vi "系统设置.vi"() -> ()   [LabVIEW 2016]
uses:
  <vilib>/Utility/miscctls.llb/LVPointTypeDef.ctl
  <vilib>/ptbypt/NI_PtbyPt.lvlib
  <vilib>/Utility/config.llb/NI_LVConfig.lvlib
panel:
  in  "多参数运行间隔":i16=4 min=0 max=24
  out "最近一次启动时间":string
  in  "站点信息设置":bool
  in  "定时重启配置":bool
  in  "模块启用配置":bool
  in  "首页显示设置":bool
  in  "开机启动":bool caption="氨氮禁用"
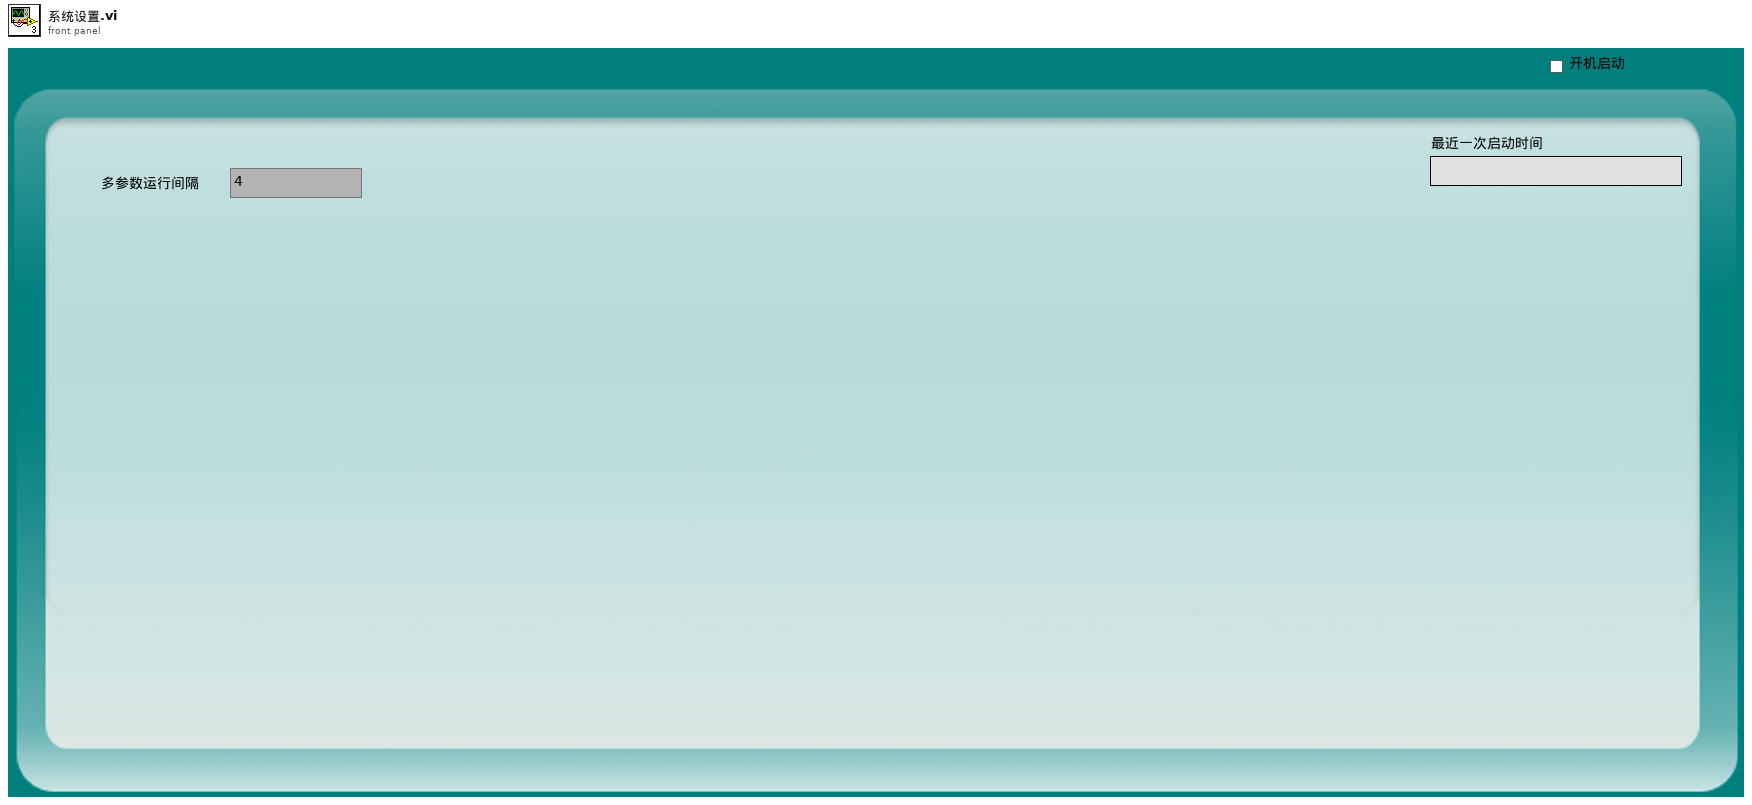
[diagram p1: front panel]
types:
  T1 = typedef "参数.ctl" = cluster{"测试模式":enum16{"水样测试", "平行样测试", "集成干预测试", "加标回收"}, "参数启用":T2}
  T2 = typedef "启动参数.ctl" = cluster{"氨氮":bool, "总磷":bool, "总氮":bool, "多参数":bool, "CODmn":bool, "CODCr":bool, "氟化物":bool, "超标留样":bool, "重金属":bool, "挥发酚":bool}
  T3 = typedef "LVPointTypeDef.ctl" = cluster{"Horizontal":i16, "Vertical":i16}
  T4 = enum8{"Enabled", "Disabled", "Disabled and Grayed Out"}
  T5 = cluster{"频次":enum16{"关闭", "每天", "星期一", "星期二", "星期三", "星期四", "星期五", "星期六", "星期日"}, "时":u16, "分":u16}
  T6 = typedef "LVDateTimeRec.ctl" = cluster{"秒数的小数部分":dbl, "秒":i32, "分":i32, "时":i32, "日":i32, "月":i32, "年":i32, "天数（周）":i32, "天数（年）":i32, "DST":i32}
  T7 = enum16{"关闭", "每天", "星期一", "星期二", "星期三", "星期四", "星期五", "星期六", "星期日"}
  T8 = typedef "NI_LVConfig.lvlib/Config Data RefNum.ctl" = refnum<k1>
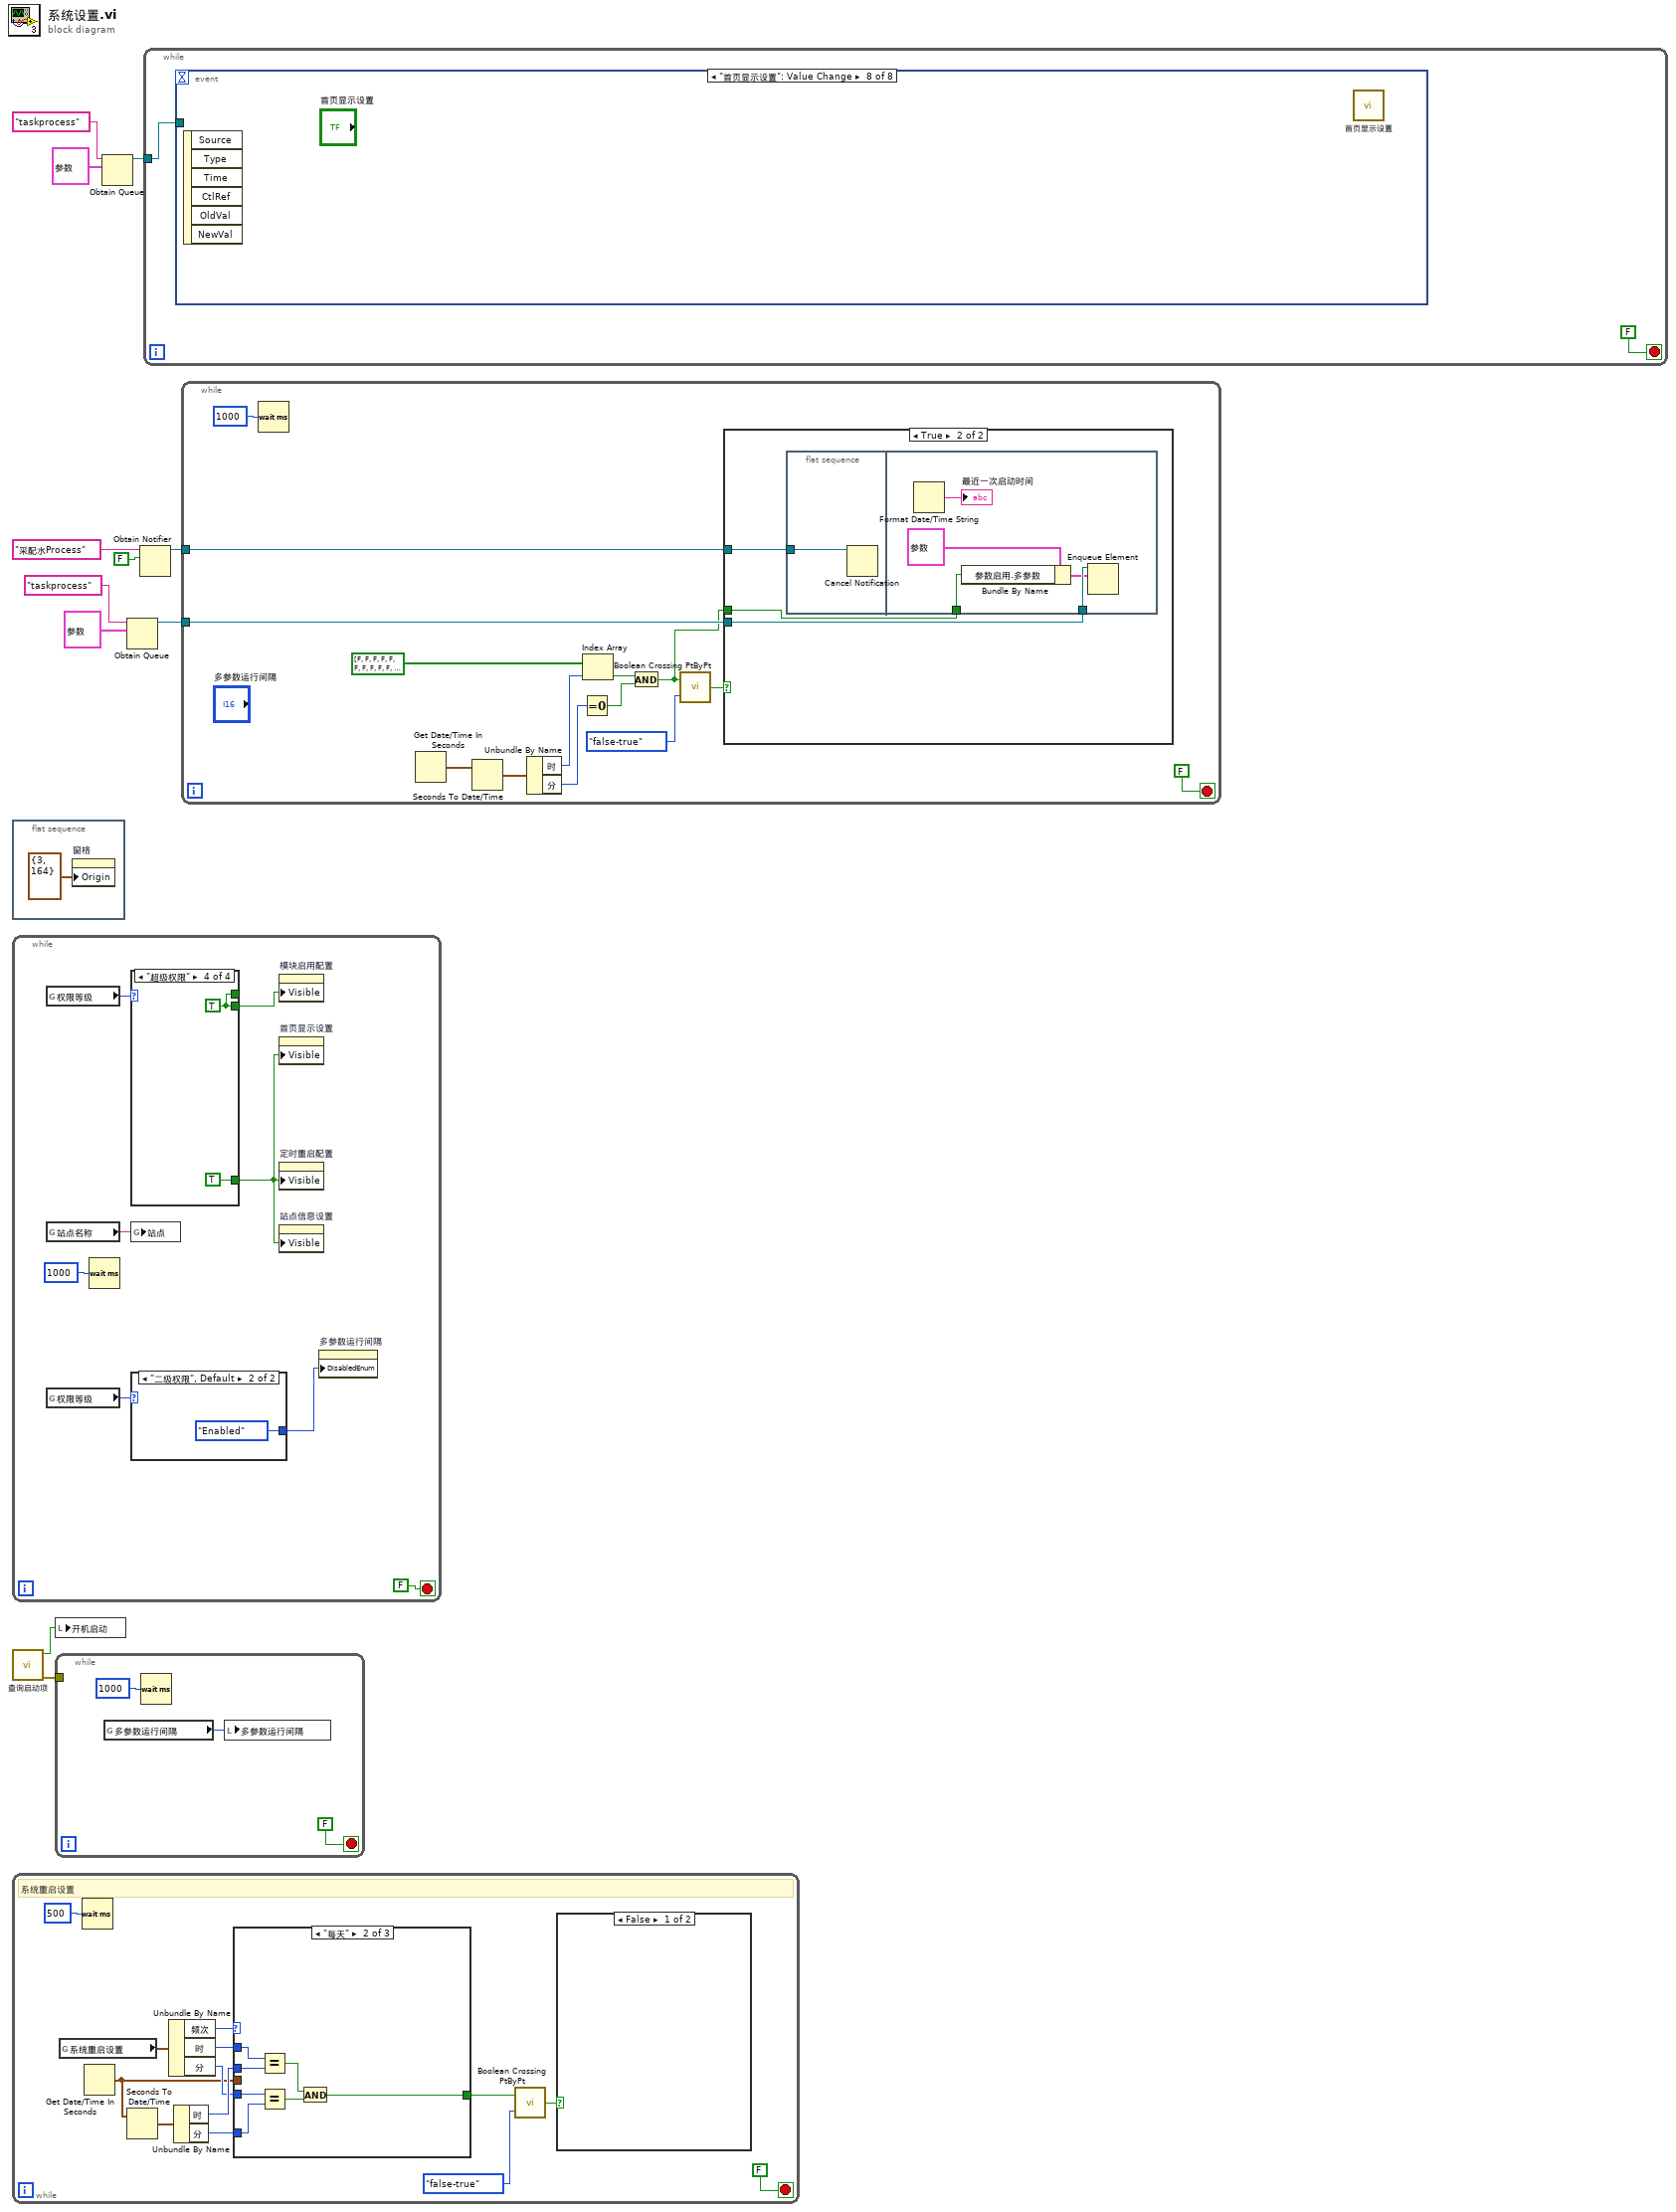
[diagram p0: block diagram]
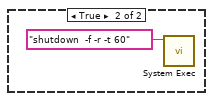
[diagram p2: hidden frame]
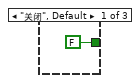
[diagram p3: hidden frame]
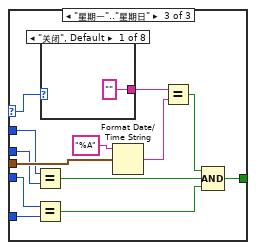
[diagram p4: hidden frame]
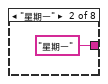
[diagram p5: hidden frame]
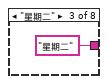
[diagram p6: hidden frame]
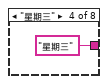
[diagram p7: hidden frame]
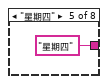
[diagram p8: hidden frame]
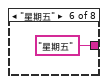
[diagram p9: hidden frame]
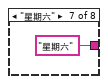
[diagram p10: hidden frame]
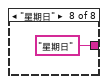
[diagram p11: hidden frame]
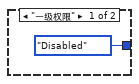
[diagram p12: hidden frame]
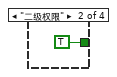
[diagram p14: hidden frame]
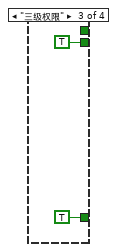
[diagram p15: hidden frame]
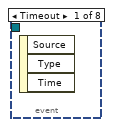
[diagram p17: hidden frame]
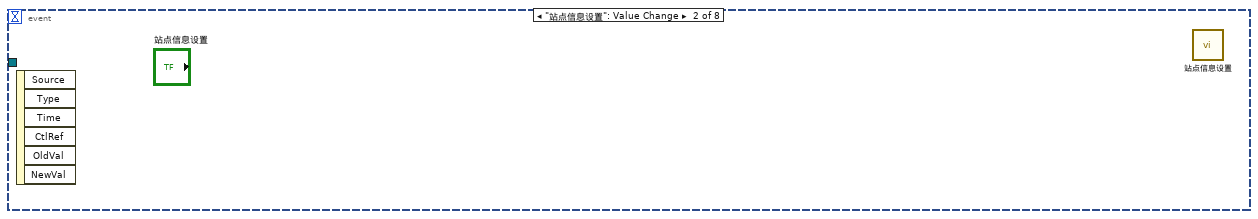
[diagram p18: hidden frame]
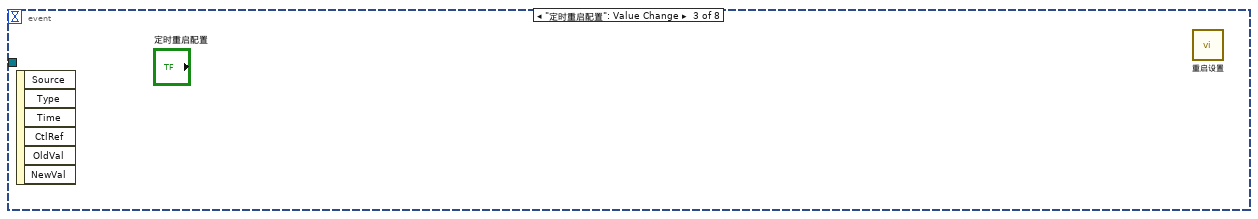
[diagram p19: hidden frame]
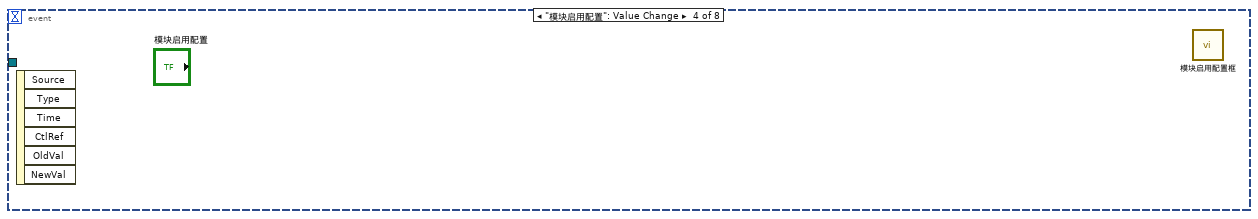
[diagram p20: hidden frame]
diagram:
  n1 = flat-sequence {
    frame #0 {
      n2 = property on="窗格" class="Pane"("Origin"=T3 {"Horizontal"=3, "Vertical"=164} ("原点")) -> ()  [unwired: 2 in, 2 out]
    }
  }
  n3 = while {
    stop <- FALSE stop-if-true
    n4 = global read "非断电保持全局变量.vi" "权限等级"() -> (w18:enum16{"一级权限", "二级权限", "三级权限", "超级权限"})
    n5 = global read "非断电保持全局变量.vi" "站点名称"() -> (w17:string)
    n6 = global read "非断电保持全局变量.vi" "权限等级"() -> (w14:enum16{"一级权限", "二级权限", "三级权限", "超级权限"})
    n7 = Wait (ms)(milliseconds to wait=u32 1000 ("等待时间（毫秒）")) -> ()  [unwired: 1 out]
    n8 = case shown="\"超级权限\"" w18 {
      tunnel: [_ TRUE TRUE TRUE] -> w15
      tunnel: [_ _ TRUE w26] -> w16
      tunnel: [_ _ _ w26] -> _
      frame "一级权限", Default {
      }
      frame "二级权限" {
      }
      frame "三级权限" {
      }
      frame "超级权限" {
        w26 = TRUE
      }
    }
    n9 = global write "短信服务全局变量.vi" "站点"(w17) -> ()
    n10 = case shown="\"二级权限\", Default" w14 {
      tunnel: [T4."Disabled" ("禁用") T4."Enabled" ("禁用")] -> w13
      frame "一级权限" {
      }
      frame "二级权限", Default {
      }
    }
    n11 = property on="模块启用配置" class="Bool"("Visible"=w16) -> ()  [unwired: 2 in, 2 out]
    n12 = property on="首页显示设置" class="Bool"("Visible"=w15) -> ()  [unwired: 2 in, 2 out]
    n13 = property on="定时重启配置" class="Bool"("Visible"=w15) -> ()  [unwired: 2 in, 2 out]
    n14 = property on="站点信息设置" class="Bool"("Visible"=w15) -> ()  [unwired: 2 in, 2 out]
    n15 = property on="多参数运行间隔" class="DigNum (strict)"("DisabledEnum"=w13) -> ()  [unwired: 2 in, 2 out]
  }
  n16 = call "查询启动项.vi"() -> ("error out"=w7:errorcluster, "包含启动项"=w8:bool)  [unwired: 10 in]
  n17 = while {
    stop <- FALSE stop-if-true
    # "系统重启设置"
    n18 = global read "系统设置全局变量.vi" "系统重启设置"() -> (w40:T5)
    n19 = Wait (ms)(milliseconds to wait=u32 500 ("等待时间（毫秒）")) -> ()  [unwired: 1 out]
    n20 = Get Date/Time In Seconds() -> (seconds since 1Jan1904=w31:timestamp)
    n21 = Seconds To Date/Time(time stamp (now)=w31) -> (date time rec=w38:T6)  [unwired: 1 in]
    n22 = Unbundle By Name(w40) -> ("频次"=w39:T7, "时"=w35:u16, "分"=w34:u16)
    n23 = Unbundle By Name(w38) -> ("时"=w37:i32, "分"=w36:i32)
    n24 = case shown="\"每天\"" w39 {
      selector: w39 -> [_ _ w60]
      tunnel: [FALSE w43 w50] -> w30
      tunnel: w37 -> [_ w49 w54]
      tunnel: w36 -> [_ w46 w52]
      tunnel: w35 -> [_ w48 w55]
      tunnel: w34 -> [_ w47 w53]
      tunnel: w31 -> [_ _ w61]
      frame "关闭", Default {
      }
      frame "每天" {
        n25 = Equal?(x=w48, y=w49) -> (x = y?=w44:bool)
        n26 = Equal?(x=w47, y=w46) -> (x = y?=w45:bool)
        n27 = And(x=w44, y=w45) -> (x .and. y?=w43:bool)
      }
      frame "星期一".."星期日" {
        n28 = Equal?(x=w55, y=w54) -> (x = y?=w56:bool)
        n29 = Equal?(x=w53, y=w52) -> (x = y?=w57:bool)
        n30 = case shown="\"关闭\", Default" w60 {
          tunnel: ["" ("时间格式字符串(%c)") "星期一" ("时间格式字符串(%c)") "星期二" ("时间格式字符串(%c)") "星期三" ("时间格式字符串(%c)") "星期四" ("时间格式字符串(%c)") "星期五" ("时间格式字符串(%c)") "星期六" ("时间格式字符串(%c)") "星期日" ("时间格式字符串(%c)")] -> w58
          frame "关闭", Default {
          }
          frame "星期一" {
          }
          frame "星期二" {
          }
          frame "星期三" {
          }
          frame "星期四" {
          }
          frame "星期五" {
          }
          frame "星期六" {
          }
          frame "星期日" {
          }
        }
        n31 = Format Date/Time String(time format string (%c)="%A" ("时间格式字符串(%c)"), seconds (now)=w61) -> (date/time string=w59:string)  [unwired: 1 in]
        n32 = Equal?(x=w58, y=w59) -> (x = y?=w51:bool)
        n33 = Compound Arithmetic op=AND ("复合运算")(w51, w56, w57) -> (w50:bool)
      }
    }
    n34 = call <vilib>:"Boolean Crossing PtByPt.vi"("direction"=enum16{"either", "false-true", "true-false"}."false-true", "input"=w30) -> ("crossing"=w28:bool)  [unwired: 1 in]
    n35 = case shown="False" w28 {
      frame False {
      }
      frame True {
        n36 = call <vilib>:"System Exec.vi"("command line"="shutdown  -f -r -t 60") -> ()  [unwired: 7 in, 4 out]
      }
    }
  }
  n37 = local write "开机启动"(w8) -> ()
  n38 = while {
    tunnel: w7 -> [_]
    stop <- FALSE stop-if-true
    n39 = global read "系统设置全局变量.vi" "多参数运行间隔"() -> (w71:i16)
    n40 = Wait (ms)(milliseconds to wait=u32 1000 ("等待时间（毫秒）")) -> ()  [unwired: 1 out]
    n41 = local write "多参数运行间隔"(w71) -> ()
  }
  n42 = Obtain Queue(name (unnamed)="taskprocess" ("名称（未命名）"), element data type=T1 {"测试模式"=enum."水样测试", "参数启用"={"氨氮"=FALSE, "总磷"=FALSE, "总氮"=FALSE, "多参数"=FALSE, "CODmn"=FALSE, "CODCr"=FALSE, "氟化物"=FALSE, "超标留样"=FALSE, "重金属"=FALSE, "挥发酚"=FALSE}} ("参数")) -> (queue out=w3:refnum<queue>)  [unwired: 3 in, 2 out]
  n43 = Obtain Queue(name (unnamed)="taskprocess" ("名称（未命名）"), element data type=T1 {"测试模式"=enum."水样测试", "参数启用"={"氨氮"=FALSE, "总磷"=FALSE, "总氮"=FALSE, "多参数"=FALSE, "CODmn"=FALSE, "CODCr"=FALSE, "氟化物"=FALSE, "超标留样"=FALSE, "重金属"=FALSE, "挥发酚"=FALSE}} ("参数")) -> (queue out=w5:refnum<queue>)  [unwired: 3 in, 2 out]
  n44 = Obtain Notifier(name (unnamed)="采配水Process" ("名称（未命名）"), notification data type=FALSE) -> (notifier out=w9:refnum<notifier>)  [unwired: 2 in, 2 out]
  n45 = while {
    tunnel: w3 -> [w74]
    stop <- FALSE stop-if-true
    n46 = event shown="[7] \"首页显示设置\": Value Change" {
      selector: _ -> [_ _ _ _ _ _ _ _]
      dyn-events: _ -> [_ _ _ _ _ _ _ _]
      timeout: _ -> [_ _ _ _ _ _ _ _]
      tunnel: w74 -> [_ _ _ _ _ _ _ _]
      event Timeout {
        n47 = event-data() -> ()  [unwired: 1 in, 3 out]
      }
      event "站点信息设置": Value Change {
        n48 = event-data() -> ()  [unwired: 1 in, 6 out]
        n49 = call "站点信息设置.vi"() -> ()  [unwired: 12 in]
      }
      event "定时重启配置": Value Change {
        n50 = event-data() -> ()  [unwired: 1 in, 6 out]
        n51 = call "重启设置.vi"() -> ()  [unwired: 12 in]
      }
      event "模块启用配置": Value Change {
        n52 = event-data() -> ()  [unwired: 1 in, 6 out]
        n53 = call "模块启用配置框.vi"() -> ()  [unwired: 12 in]
      }
      event "多参数运行间隔": Value Change {
        n54 = event-data() -> ()  [unwired: 1 in, 6 out]
        n55 = flat-sequence {
          frame #0 {
          }
          frame #1 {
            n56 = local read "多参数运行间隔"() -> (w76:i16)
            n57 = global write "系统设置全局变量.vi" "多参数运行间隔"(w76) -> ()
          }
          frame #2 {
            n58 = call <vilib>:"Application Directory.vi"() -> ("Application Directory"=w90:path)
            n59 = Build Path(base path=w90, name or relative path="data\\sys.ini" ("名称或相对路径")) -> (appended path=w88:path)
            n60 = call <vilib>:"Open Config Data.vi"("configuration file path"=w88) -> ("error out"=w84:errorcluster, "refnum"=w87:T8)  [unwired: 8 in, 1 out]
            n61 = vi-ref "系统设置全局变量.vi"() -> (w86:refnum<vi>)
            n62 = call <userlib>:"Write Panel to INI__ogtk.vi"("error in (no error)"=w84, "VI ref"=w86, "refnum"=w87) -> ("error out"=w83:errorcluster, "refnum out"=w85:T8)  [unwired: 7 in]
            n63 = call <vilib>:"Close Config Data.vi"("error in (no error)"=w83, "refnum"=w85) -> ("error out"=w78:errorcluster, "file path"=w77:path)  [unwired: 8 in]
            n64 = Open/Create/Replace File(file path (use dialog)=w77, error in=w78) -> (refnum out=w81:refnum<file>, error out=w82:errorcluster)  [unwired: 4 in, 1 out]
            n65 = Flush File(refnum=w81, error in=w82) -> (refnum out=w80:refnum<file>, error out=w79:errorcluster)
            n66 = Close File(refnum=w80, error in=w79) -> ()  [unwired: 2 out]
          }
        }
      }
      event "多参数运行间隔": Mouse Down {
        n67 = event-data() -> ("CtlRef"=w93:refnum<vi>)  [unwired: 1 in, 7 out]
        n68 = property class="DigNum (strict)"(reference=w93) -> (reference out=w92:refnum<vi>, "DisabledEnum"=w91:T4)  [unwired: 1 in, 1 out]
        n69 = case shown="\"Enabled\", Default" w91 {
          tunnel: w92 -> [w94 _]
          frame "Enabled", Default {
            n70 = property class="DigNum (strict)"(reference=w94) -> (reference out=w97:refnum<vi>, "Value"=w96:i16)  [unwired: 1 in, 1 out]
            n71 = call "数字键盘.vi"("OldNumber"=w96) -> ("NewNumber"=w95:sgl)
            n72 = property class="DigNum (strict)"(reference=w97, "Val(Sgnl)"=w95) -> ()  [unwired: 1 in, 2 out]
          }
          frame "Disabled" {
            n73 = One Button Dialog(message="权限不足，请提升操作权限！" ("消息")) -> ()  [unwired: 1 in, 1 out]
          }
        }
      }
      event "开机启动": Value Change {
        n74 = event-data() -> ("NewVal"=w99:bool)  [unwired: 1 in, 5 out]
        n75 = case shown="False" w99 {
          frame False {
            n76 = call "删除启动项.vi"() -> ("删除标记"=w100:bool)  [unwired: 10 in, 1 out]
            n77 = case shown="False" w100 {
              frame False {
                n78 = local write "开机启动"(TRUE ("开机启动")) -> ()
                n79 = One Button Dialog(message="启动项删除失败" ("消息")) -> ()  [unwired: 1 in, 1 out]
              }
              frame True {
              }
            }
          }
          frame True {
            n80 = call "添加启动项.vi"() -> ("添加成功标记"=w103:bool)  [unwired: 10 in, 1 out]
            n81 = case shown="False" w103 {
              frame False {
                n82 = local write "开机启动"(FALSE ("开机启动")) -> ()
                n83 = One Button Dialog(message="启动项添加失败" ("消息")) -> ()  [unwired: 1 in, 1 out]
              }
              frame True {
              }
            }
          }
        }
      }
      event "首页显示设置": Value Change {
        n84 = event-data() -> ()  [unwired: 1 in, 6 out]
        n85 = call "首页显示设置.vi"() -> ()  [unwired: 12 in]
      }
    }
  }
  n86 = while {
    tunnel: w9 -> [w117]
    tunnel: w5 -> [w115]
    stop <- FALSE stop-if-true
    n87 = Wait (ms)(milliseconds to wait=u32 1000 ("等待时间（毫秒）")) -> ()  [unwired: 1 out]
    n88 = Get Date/Time In Seconds() -> (seconds since 1Jan1904=w113:timestamp)
    n89 = Seconds To Date/Time(time stamp (now)=w113) -> (date time rec=w112:T6)  [unwired: 1 in]
    n90 = Unbundle By Name(w112) -> ("时"=w109:i32, "分"=w111:i32)
    n91 = Equal To 0?(x=w111) -> (x = 0?=w110:bool)
    n92 = Index Array(array=bool[] [FALSE, FALSE, FALSE, FALSE, FALSE, FALSE, FALSE, FALSE, FALSE, FALSE, FALSE, FALSE, FALSE, FALSE, FALSE, FALSE, FALSE, FALSE, FALSE, FALSE, FALSE, FALSE, FALSE, FALSE] ("24H周期设置"), index=w109) -> (element=w108:bool)
    n93 = And(x=w108, y=w110) -> (x .and. y?=w107:bool)
    n94 = call <vilib>:"Boolean Crossing PtByPt.vi"("direction"=enum16{"either", "false-true", "true-false"}."false-true", "input"=w107) -> ("crossing"=w114:bool)  [unwired: 1 in]
    n95 = case shown="True" w114 {
      tunnel: w117 -> [_ w122]
      tunnel: w107 -> [_ w121]
      tunnel: w115 -> [_ w120]
      frame False {
      }
      frame True {
        n96 = flat-sequence {
          tunnel: w122 -> [w123]
          tunnel: w121 -> [w124]
          tunnel: w120 -> [w128]
          frame #0 {
            n97 = Cancel Notification(0:w123) -> ()  [unwired: 1 in, 3 out]
          }
          frame #1 {
            n98 = Format Date/Time String() -> (date/time string=→"最近一次启动时间":string)  [unwired: 3 in]
            n99 = Bundle By Name(cluster=T1 {"测试模式"=enum."水样测试", "参数启用"={"氨氮"=FALSE, "总磷"=FALSE, "总氮"=FALSE, "多参数"=FALSE, "CODmn"=FALSE, "CODCr"=FALSE, "氟化物"=FALSE, "超标留样"=FALSE, "重金属"=FALSE, "挥发酚"=FALSE}} ("参数"), "参数启用.多参数"=w124) -> (w127:T1)
            n100 = Enqueue Element(queue=w128, element=w127) -> ()  [unwired: 2 in, 3 out]
          }
        }
      }
    }
  }
